vi "Yokogawa - take measurement.vi"(8 "error in":errorcluster, 9 "UI":refnum<queue>, 11 "Hardware Resources in":T1={"VISA resource name"="", "Mode (0: Normal) "=0, "Voltage"={"Element (0: All)"=0, "V Range (200)"=4}, "Current"={"A Range (2)"=7, "A Terminal (0: 5A)"=0, "Element (0: ALL)"=0}, "Observation Time"=10, "Modules on/off"={"Module 1"=FALSE, "Module 2"=FALSE, "Module 3"=FALSE, "Module 4"=FALSE}} {"Observation Time" items=["1ksec", "400sec", "200sec", "100sec", "40sec", "20sec", "10sec", "4sec", "2sec", "1sec", "400msec", "200msec", "100msec", "40msec", "20msec", "10msec", "4msec", "2msec", "1msec", "400usec", "200usec", "100usec", "40usec", "20usec", "10usec"]; "Mode (0: Normal)" items=["Normal", "Harmonics"]; "Current"."Element (0: ALL)" items=["All", "Element 1", "Element 2", "Element 3", "Element 4"]; "Current"."A Terminal (0: 5A)" items=["5A", "20A", "Sensor"]; "Current"."A Range (2)" items=["AUTO", "0.1", "0.2", "0.4", "1", "2", "4", "10", "20", "40", "100"]; "Voltage"."V Range (200)" items=["AUTO", "30", "60", "120", "200", "300", "600", "1200", "2000"]; "Voltage"."Element (0: All)" items=["All", "Element 1", "Element 2", "Element 3", "Element 4"]}) -> (0 "error out":errorcluster, 3 "Electrical Data":T2={"Time Stamp"=timestamp(0 s since 1904-01-01), "Temperature (C)"=0.0, "Electrical Data"=[["   NaN", "   NaN", "   NaN", "   NaN"], ["   NaN", "   NaN", "   NaN", "   NaN"], ["   NaN", "   NaN", "   NaN", "   NaN"], ["   NaN", "   NaN", "   NaN", "   NaN"], ["   NaN", "   NaN", "   NaN", "   NaN"], ["   NaN", "   NaN", "   NaN", "   NaN"], ["   NaN", "   NaN", "   NaN", "   NaN"], ["   NaN", "   NaN", "   NaN", "   NaN"], ["   NaN", "   NaN", "   NaN", "   NaN"], ["   NaN", "   NaN", "   NaN", "   NaN"]], "Waveform Graph"=[]})   [LabVIEW 2014, in "Yokogawa.lvlib" / "YKPZ400 Acquisition.lvlib"]
doc: "Take normal measurements, harmonic measurements, and collect waveforms"
uses:
  YKPZ400 Acquisition.lvlib
  controls/electrical2.ctl
  Hardware Configuration.ctl
  support/Message Queue/Message Cluster.ctl
  support/Message Queue/Enqueue Message (Single).vi
  Libraries/Yokogawa PZ4000/Yokogawa PZ4000.lvlib
  support/Message Queue/YKPZ400 Message Queue.lvlib
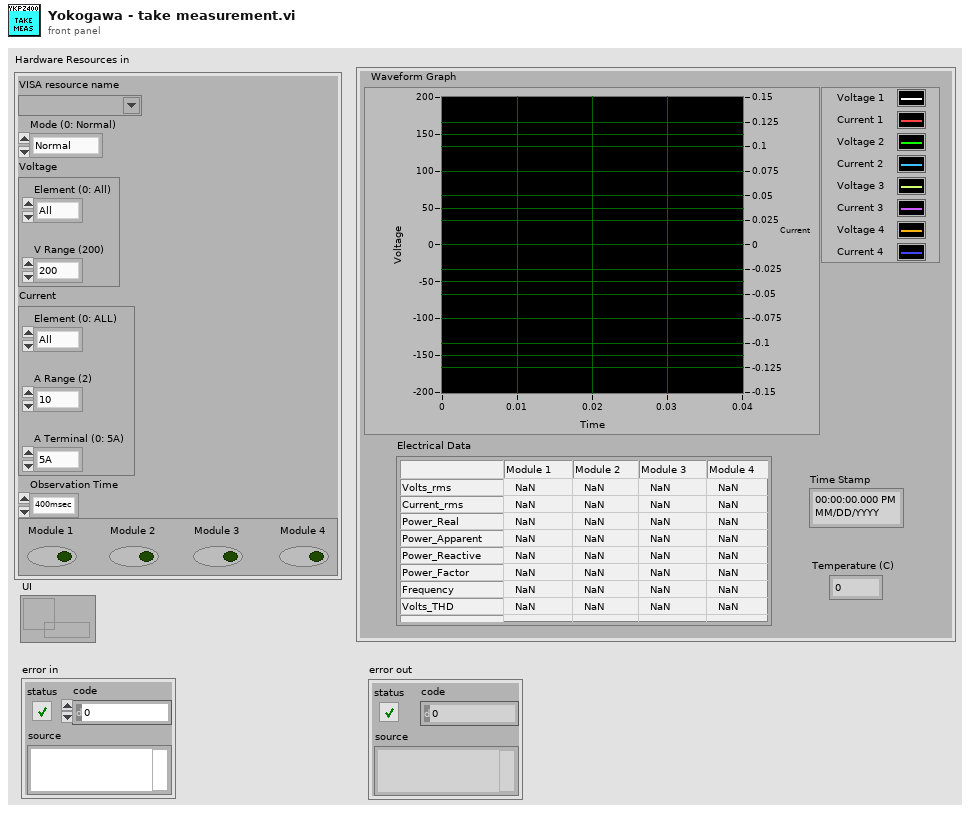
[diagram p1: front panel]
types:
  T1 = typedef "Yokogawa.lvlib/YKPZ400 Acquisition.lvlib/Hardware Configuration.ctl" = cluster{"VISA resource name":refnum<visa-resource-name>, "Mode (0: Normal) ":u16, "Voltage":cluster{"Element (0: All)":u16, "V Range (200)":u16}, "Current":cluster{"A Range (2)":u16, "A Terminal (0: 5A)":u16, "Element (0: ALL)":u16}, "Observation Time":u16, "Modules on/off":cluster{"Module 1":bool, "Module 2":bool, "Module 3":bool, "Module 4":bool}}
  T2 = typedef "Yokogawa.lvlib/YKPZ400 Acquisition.lvlib/electrical2.ctl" = cluster{"Time Stamp":timestamp, "Temperature (C)":dbl, "Electrical Data":string[][], "Waveform Graph":waveform(dbl)[]}
  T3 = cluster{"Module 1":bool, "Module 2":bool, "Module 3":bool, "Module 4":bool}
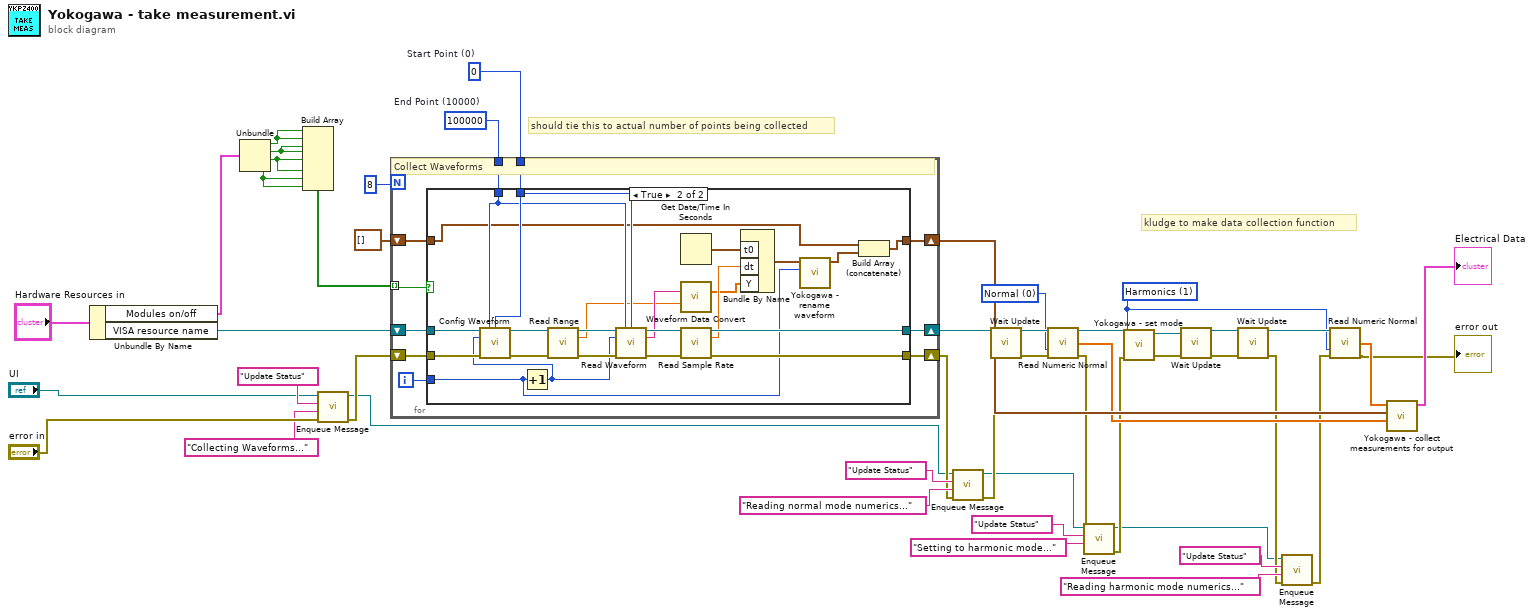
[diagram p0: block diagram]
diagram:
  w47 = u32 100000  # End Point (10000)
  w48 = u32 0  # Start Point (0)
  w27 = u16 1 items=["Normal", "Harmonics"] ("Mode (0: Normal)  2")
  w33 = u16 0 items=["Normal", "Harmonics"] ("Mode (0: Normal)")
  # "should tie this to actual number of points being collected"
  # "kludge to make data collection function"
  n1 = Unbundle By Name("Hardware Resources in") -> ("Modules on/off"=w23:T3, "VISA resource name"=w22:refnum<visa-resource-name>)
  n2 = Unbundle(w23) -> ("Module 1"=w44:bool, "Module 2"=w43:bool, "Module 3"=w42:bool, "Module 4"=w41:bool)
  n3 = Build Array(w44, w44, w43, w43, w42, w42, w41, w41) -> (w45:bool[])
  n4 = call-poly "Enqueue Message.vi"("error in (no error)"="error in", "Message Data"="Collecting Waveforms..." ("Message"), "Message"="Update Status", "Message Queue"="UI") -> ("error out"=w18:errorcluster, "dup Message Queue"=w3:refnum<queue>)  [unwired: 6 in]
  n5 = for {
    N: 8 -> [_]
    tunnel: w48 -> [w58]
    tunnel: w47 -> [w57]
    shift-right: [w54] -> w36
    shift-left: w22 -> [w56]
    shift-right: [w53] -> w9
    shift-left: w18 -> [w55]
    shift-right: [w51] -> w39
    shift-left: waveform(dbl)[] [] -> [w50]
    tunnel: w45 -> [w49] mode=indexing
    i -> [w52]
    # "Collect Waveforms"
    n6 = case shown="True" w49 {
      tunnel: w58 -> [_ w84]
      tunnel: w57 -> [_ w81]
      tunnel: w56 -> [w60 w79]
      tunnel: w55 -> [w59 w78]
      tunnel: [w60 w74] -> w54
      tunnel: [w59 w73] -> w53
      tunnel: w52 -> [_ w62]
      tunnel: [w61 w71] -> w51
      tunnel: w50 -> [w61 w70]
      frame False {
      }
      frame True {
        n7 = Increment(x=w62) -> (x+1=w63:i32)
        n8 = call "Config Waveform.vi"("VISA resource name"=w79, "End Point (1000)"=w81, "Start Point (0)"=w84, "Select Trace (1)"=w63, "error in (no error)"=w78) -> ("VISA resource name out"=w77:refnum<visa-resource-name>, "error out"=w82:errorcluster)  [unwired: 9 in]
        n9 = call "Read Range.vi"("VISA resource name"=w77, "error in (no error)"=w82) -> ("VISA resource name out"=w76:refnum<visa-resource-name>, "Range"=w69:dbl, "error out"=w80:errorcluster)  [unwired: 11 in]
        n10 = call "Read Waveform.vi"("VISA resource name"=w76, "End Point (1000)"=w81, "Start Point (0)"=w84, "Select Trace (1)"=w63, "error in (no error)"=w80) -> ("VISA resource name out"=w75:refnum<visa-resource-name>, "Waveform Data"=w72:string, "error out"=w83:errorcluster)  [unwired: 8 in]
        n11 = Get Date/Time In Seconds() -> (seconds since 1Jan1904=w66:timestamp)
        n12 = call "Waveform Data Convert.vi"("Input Data"=w72, "Range"=w69) -> ("Output"=w67:dbl[])  [unwired: 11 in, 2 out]
        n13 = call "Read Sample Rate.vi"("VISA resource name"=w75, "error in (no error)"=w83) -> ("VISA resource name out"=w74:refnum<visa-resource-name>, "Delta T"=w68:dbl, "error out"=w73:errorcluster)  [unwired: 11 in]
        n14 = Bundle By Name("t0"=w66, "dt"=w68, "Y"=w67) -> (w65:waveform(dbl))  [unwired: 1 in]
        n15 = call "Yokogawa - rename waveform.vi"("Itteration"=w62, "Waveform in"=w65) -> ("Waveform out"=w64:waveform(dbl))  [unwired: 9 in]
        n16 = Build Array (concatenate)(w70, w64) -> (w71:waveform(dbl)[])
      }
    }
  }
  n17 = call-poly "Enqueue Message.vi"("error in (no error)"=w9, "Message Data"="Reading normal mode numerics..." ("Message"), "Message"="Update Status", "Message Queue"=w3) -> ("error out"=w8:errorcluster, "dup Message Queue"=w2:refnum<queue>)  [unwired: 6 in]
  n18 = call "Wait Update.vi"("VISA resource name"=w36, "error in (no error)"=w8) -> ("VISA resource name out"=w37:refnum<visa-resource-name>, "error out"=w38:errorcluster)  [unwired: 12 in]
  n19 = call "Read Numeric Normal.vi"("VISA resource name"=w37, "Mode (0: Normal)"=w33, "error in (no error)"=w38) -> ("VISA resource name out"=w34:refnum<visa-resource-name>, "Measure"=w35:dbl[], "error out"=w7:errorcluster)  [unwired: 9 in, 1 out]
  n20 = call-poly "Enqueue Message.vi"("error in (no error)"=w7, "Message Data"="Setting to harmonic mode..." ("Message"), "Message"="Update Status", "Message Queue"=w2) -> ("error out"=w6:errorcluster, "dup Message Queue"=w1:refnum<queue>)  [unwired: 6 in]
  n21 = call "Yokogawa - set mode.vi"("error in (no error)"=w6, "Mode (0: Normal)"=w27, "VISA Refnum in"=w34) -> ("error out"=w28:errorcluster, "VISA Refnum out"=w31:refnum<visa-resource-name>)  [unwired: 7 in]
  n22 = call "Wait Update.vi"("VISA resource name"=w31, "error in (no error)"=w28) -> ("VISA resource name out"=w30:refnum<visa-resource-name>, "error out"=w29:errorcluster)  [unwired: 12 in]
  n23 = call "Wait Update.vi"("VISA resource name"=w30, "error in (no error)"=w29) -> ("VISA resource name out"=w32:refnum<visa-resource-name>, "error out"=w5:errorcluster)  [unwired: 12 in]
  n24 = call-poly "Enqueue Message.vi"("error in (no error)"=w5, "Message Data"="Reading harmonic mode numerics..." ("Message"), "Message"="Update Status", "Message Queue"=w1) -> ("error out"=w4:errorcluster)  [unwired: 6 in, 1 out]
  n25 = call "Read Numeric Normal.vi"("VISA resource name"=w32, "Mode (0: Normal)"=w27, "error in (no error)"=w4) -> ("Measure"=w26:dbl[], "error out"=→"error out":errorcluster)  [unwired: 9 in, 2 out]
  n26 = call "Yokogawa - collect measurements for output.vi"("Normal Measurements"=w35, "Waveforms In"=w39, "Harmonic Measurements"=w26) -> ("Electrical Data Out"=→"Electrical Data":T2)  [unwired: 8 in]
